vi "Normalize String - String with Invalid Character - Normalized String does not contain Invalid Character.vi"() -> ()   [LabVIEW 2013, in "JUnit XML Tests.lvlib"]
uses:
  JUnit XML Tests.lvlib
  <vilib>/addons/_JKI Toolkits/Caraya/classes/Assert/Assert Equal Value_Variant.vi
  <vilib>/addons/_JKI Toolkits/Caraya/classes/Test/Test.lvclass
  JUnit XML/JUnit XML.lvlib
  <vilib>/addons/_JKI Toolkits/Caraya/classes/Assert/Assert.lvclass
panel:
  out "error out":errorcluster
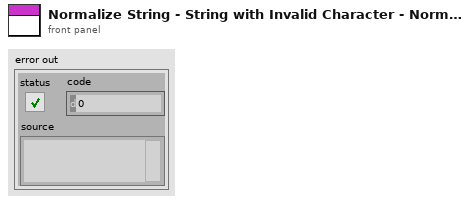
[diagram p1: front panel]
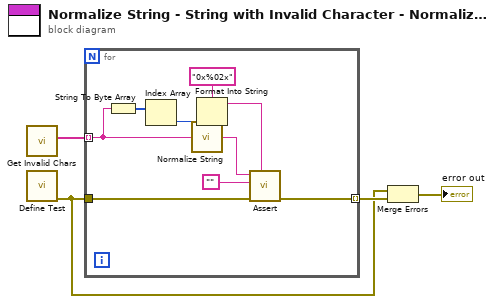
[diagram p0: block diagram]
diagram:
  n1 = call "Get Invalid Chars.vi"() -> ("invalid chars"=w4:string[])  [unwired: 11 in]
  n2 = call <vilib>:"Define Test.vi"() -> ("error out"=w2:errorcluster)  [unwired: 10 in, 1 out]
  n3 = for {
    tunnel: w2 -> [w13]
    tunnel: w4 -> [w5] mode=indexing
    tunnel: [w10] -> w3 mode=indexing
    n4 = String To Byte Array(string=w5) -> (unsigned byte array=w7:u8[])
    n5 = Index Array(array=w7) -> (element=w8:u8)  [unwired: 1 in]
    n6 = call "Normalize String.vi"("String"=w5) -> ("Normalized String"=w12:string)  [unwired: 1 in]
    n7 = Format Into String(format string="0x%02x", w8) -> (resulting string=w6:string)  [unwired: 2 in, 1 out]
    n8 = call-poly <vilib>:"Assert.vi"("Label"=w6, "error in (no error)"=w13, "Actual"="", "Expected"=w12) -> ("error out"=w10:errorcluster)  [unwired: 6 in, 1 out]
  }
  n9 = Merge Errors(w2, w3) -> (→"error out":errorcluster)
